vi "timing_data_to_boolean_array.vi"(2 "end time [s]":dbl=1.0, 3 "start time [s]":dbl, 4 "overall length [s]":dbl=1000.0) -> (0 "boolean timing array":bool[](array[boolean]))   [LabVIEW 2012]
doc: "Creates a boolean array based on the timing info send in. Used to display a digital waveform graph to visualize the timing info recieved and send to the Standford Research Systems DG645 Delay Generator. \nWorks only in combination with values in seconds. Can be used for any timing value in combination with the standardize array vi."
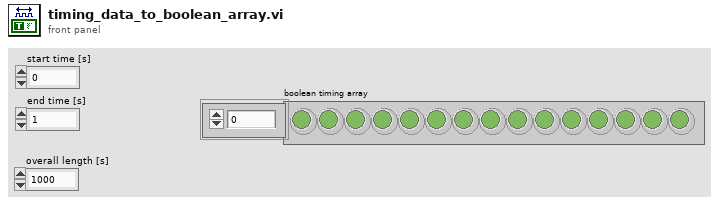
[diagram p1: front panel]
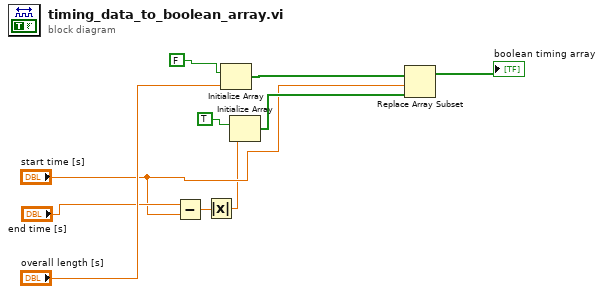
[diagram p0: block diagram]
diagram:
  n1 = Subtract(x="end time [s]", y="start time [s]") -> (x-y=w4:dbl)
  n2 = Absolute Value(x=w4) -> (abs(x)=w1:dbl)
  n3 = Initialize Array(FALSE, "overall length [s]") -> (w8:bool[])
  n4 = Initialize Array(TRUE ("new element/subarray"), w1) -> (w6:bool[])
  n5 = Replace Array Subset(array=w8, new element=w6, index="start time [s]") -> (→"boolean timing array":bool[])
